vi "Read VI Ref.vi"(8 "error in (no error)":errorcluster, 11 "TestEngineReference in":refnum<class "TestEngineReference.lvclass">) -> (0 "error out":errorcluster, 2 "VI Ref":refnum<vi>, 3 "TestEngineReference out":refnum<class "TestEngineReference.lvclass">)   [LabVIEW 2019, in "TestEngine.lvlib" / "TestEngineReference.lvclass"]
uses:
  TestEngineReference.lvclass
  TestEngineReference.lvclass/TestEngineReference.ctl
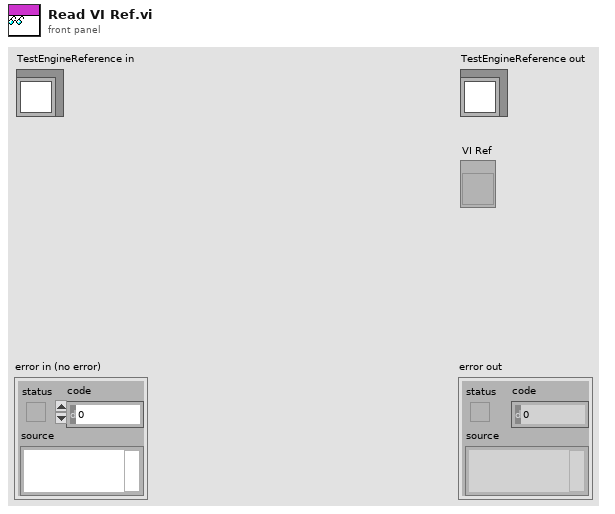
[diagram p1: front panel]
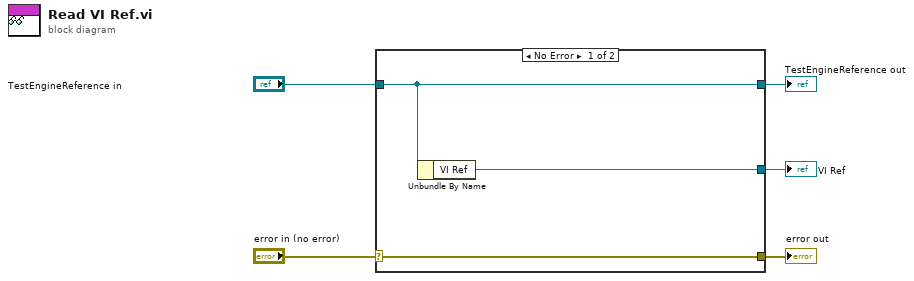
[diagram p0: block diagram]
diagram:
  n1 = case shown="No Error" "error in (no error)" {
    selector: "error in (no error)" -> [w8 w9]
    tunnel: [w8 w9] -> w4
    tunnel: [w7 w10] -> w2
    tunnel: "TestEngineReference in" -> [w7 w10]
    tunnel: [w6 _] -> w1
    frame No Error {
      n2 = Unbundle By Name(w7) -> ("VI Ref"=w6:refnum<vi>)
    }
    frame Error {
    }
  }
  "error out" <- w4
  "TestEngineReference out" <- w2
  "VI Ref" <- w1
